vi "Coord window-Delete coordinates.vi"(10 "Do not check key focus":bool) -> (0 "error out":errorcluster)   [LabVIEW 2020]
uses:
  Globals/Coord window-Globals.vi
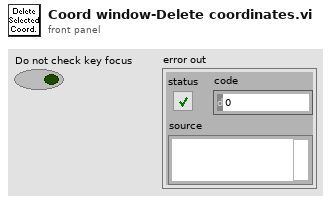
[diagram p1: front panel]
types:
  T1 = typedef "Coordinate list window refs.ctl" = cluster{"Window Name (i.e. Key)":string, "menu reference":refnum<k9>, "VI's reference":refnum<vi>, "Pane 1":refnum<vi>, "Pane 2":refnum<vi>, "Coord Listbox":refnum<vi>, "File name":refnum<vi>, "Picture Map":refnum<vi>, "Stage XYZ Position ind.":refnum<vi>}
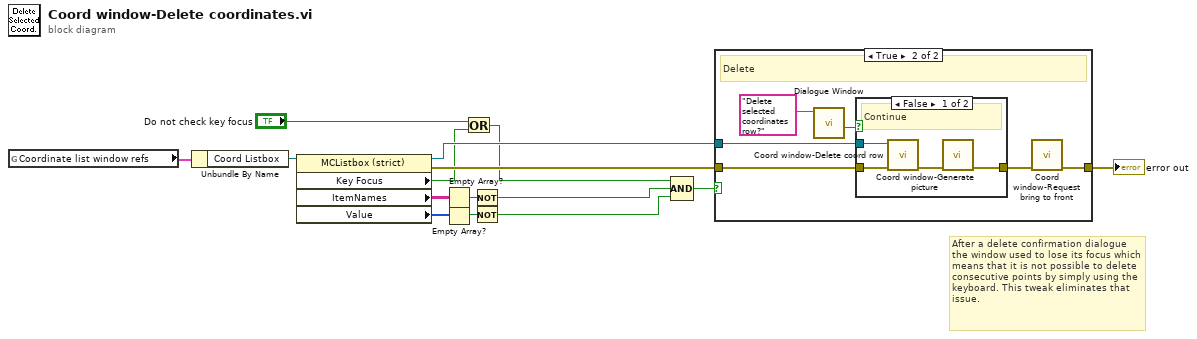
[diagram p0: block diagram]
diagram:
  # "After a delete confirmation dialogue the window used to lose its focus which means that it is not possible to delete consecutive points by simply using the keyboard. This tweak eliminates that issue."
  n1 = global read "Coord window-Globals.vi" "Coordinate list window refs"() -> (w15:T1)
  n2 = Unbundle By Name(w15) -> ("Coord Listbox"=w5:refnum<vi>)
  n3 = property on="Property Node" class="MCListbox (strict)"(reference=w5) -> (reference out=w12:refnum<vi>, error out=w13:errorcluster, "Key Focus"=w2:bool, "ItemNames"=w4:string[][], "Value"=w8:i32[])  [unwired: 1 in]
  n4 = Empty Array?(array=w4) -> (empty?=w6:bool)
  n5 = Empty Array?(array=w8) -> (empty?=w9:bool)
  n6 = Or(x="Do not check key focus", y=w2) -> (x .or. y?=w1:bool)
  n7 = Not(x=w6) -> (.not. x?=w7:bool)
  n8 = Not(x=w9) -> (.not. x?=w10:bool)
  n9 = Compound Arithmetic op=AND(w1, w7, w10) -> (w11:bool)
  n10 = case shown="True" w11 {
    tunnel: w12 -> [_ w22]
    tunnel: w13 -> [w16 w21]
    tunnel: [w16 w17] -> w14
    frame False {
      # "Ignore"
    }
    frame True {
      # "Delete"
      n11 = call "Dialogue Window.vi"("Message string"="Delete selected coordinates row?") -> ("Cancelled (Left button pressed)"=w19:bool)  [unwired: 8 in, 2 out]
      n12 = case shown="False" w19 {
        tunnel: w22 -> [w26 _]
        tunnel: w21 -> [w25 w27]
        tunnel: [w23 w27] -> w18
        frame False {
          # "Continue"
          n13 = call "Coord window-Delete coord row.vi"("error in (no error)"=w25, "MulticolumnListbox in"=w26) -> ("error out"=w24:errorcluster)  [unwired: 8 in, 1 out]
          n14 = call "Coord window-Generate picture.vi"("error in (no error)"=w24) -> ("error out"=w23:errorcluster)  [unwired: 10 in]
        }
        frame True {
          # "Cancelled"
        }
      }
      n15 = call "Coord window-Request bring to front.vi"("error in (no error)"=w18) -> ("error out"=w17:errorcluster)  [unwired: 10 in]
    }
  }
  "error out" <- w14
